vi "Write CMD.vi"(8 "error in (no error)":errorcluster, 10 "CMD":refnum<class "Command.lvclass">, 11 "Forward Command MSG in":refnum<class "Forward Command MSG.lvclass">) -> (0 "error out":errorcluster, 3 "Forward Command MSG out":refnum<class "Forward Command MSG.lvclass">)   [LabVIEW 2017, in "Controller.lvlib" / "Forward Command MSG.lvclass"]
uses:
  Forward Command MSG.lvclass
  <vilib>/MSR Consulting, LLC/General Reuse/Command/Command.lvclass
  Forward Command MSG.lvclass/Forward Command MSG.ctl
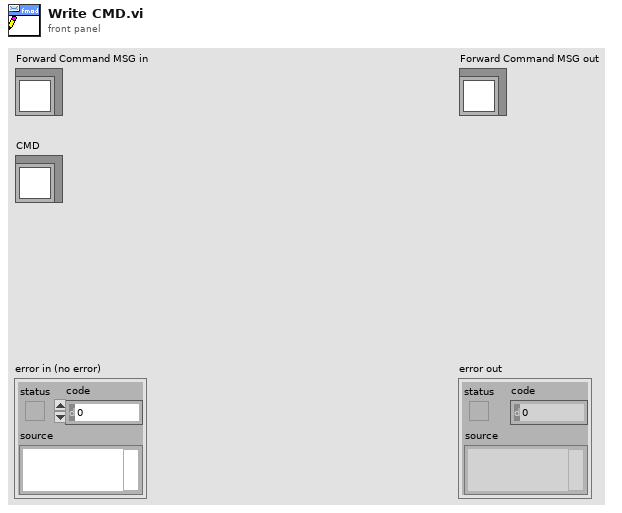
[diagram p1: front panel]
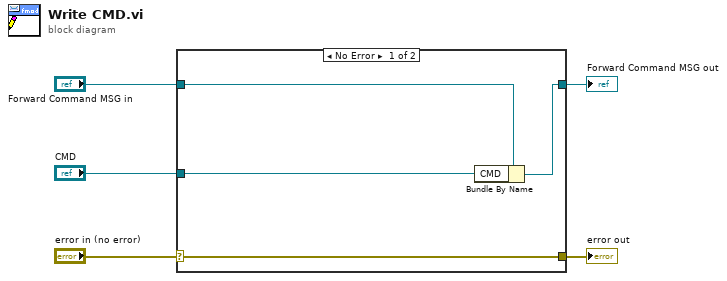
[diagram p0: block diagram]
diagram:
  n1 = case shown="No Error" "error in (no error)" {
    selector: "error in (no error)" -> [w9 w10]
    tunnel: [w9 w10] -> w4
    tunnel: [w7 w11] -> w2
    tunnel: "Forward Command MSG in" -> [w8 w11]
    tunnel: "CMD" -> [w6 _]
    frame No Error {
      n2 = Bundle By Name(cluster=w8, "CMD"=w6) -> (w7:refnum<class "Forward Command MSG.lvclass">)
    }
    frame Error {
    }
  }
  "error out" <- w4
  "Forward Command MSG out" <- w2
